vi "AO_Volt_and_Curr.vi"(6 "Curnt_Value":dbl[](array[numeric]) format="%0.2f", 7 "Volt_Value":dbl[](array[numeric]) format="%0.2f", 9 "Current Channel":string[](array[string]), 10 "Volt Channel":string[](array[string])) -> (0 "error out":errorcluster)   [LabVIEW 2017]
uses:
  <vilib>/DAQmx/write.llb/DAQmx Write (Analog 1D DBL NChan 1Samp).vi
  <vilib>/DAQmx/create/channels.llb/DAQmx Create Channel (AO-Voltage-Basic).vi
  <vilib>/DAQmx/miscellaneous.llb/DAQmx Fill In Error Info.vi
  <vilib>/DAQmx/create/channels.llb/DAQmx Create Channel (AO-Current-Basic).vi
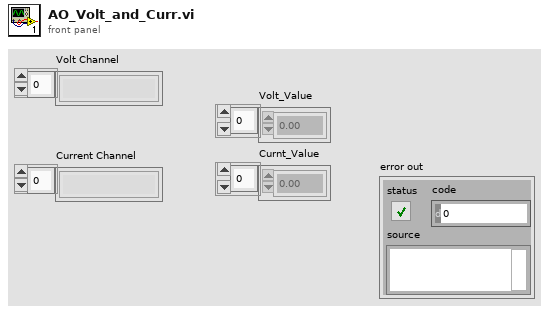
[diagram p1: front panel]
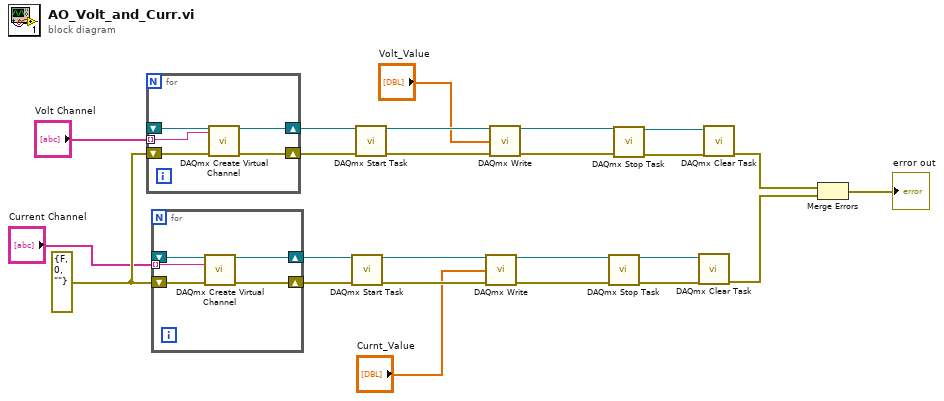
[diagram p0: block diagram]
diagram:
  w4 = errorcluster {"status"=FALSE, "code"=0, "source"=""} ("error out")
  n1 = for {
    shift-right: [w29] -> w24
    shift-left: _ -> [w27]
    shift-right: [w28] -> w23
    shift-left: w4 -> [w26]
    tunnel: "Volt Channel" -> [w25] mode=indexing
    n2 = call-poly <vilib>:"DAQmx Create Virtual Channel.vi"("task in"=w27, "physical channels"=w25, "error in"=w26) -> ("task out"=w29:refnum<k21>, "error out"=w28:errorcluster)  [unwired: 11 in]
  }
  n3 = for {
    shift-right: [w34] -> w18
    shift-left: _ -> [w32]
    shift-right: [w33] -> w17
    shift-left: w4 -> [w31]
    tunnel: "Current Channel" -> [w30] mode=indexing
    n4 = call-poly <vilib>:"DAQmx Create Virtual Channel.vi"("task in"=w32, "physical channels"=w30, "error in"=w31) -> ("task out"=w34:refnum<k21>, "error out"=w33:errorcluster)  [unwired: 11 in]
  }
  n5 = call <vilib>:"DAQmx Start Task.vi"("task/channels in"=w18, "error in"=w17) -> ("task out"=w19:refnum<k21>, "error out"=w20:errorcluster)  [unwired: 12 in]
  n6 = call <vilib>:"DAQmx Start Task.vi"("task/channels in"=w24, "error in"=w23) -> ("task out"=w22:refnum<k21>, "error out"=w21:errorcluster)  [unwired: 12 in]
  n7 = call-poly <vilib>:"DAQmx Write.vi"("task/channels in"=w19, "data"="Curnt_Value", "error in"=w20) -> ("task out"=w10:refnum<k21>, "error out"=w9:errorcluster)  [unwired: 10 in, 1 out]
  n8 = call-poly <vilib>:"DAQmx Write.vi"("task/channels in"=w22, "data"="Volt_Value", "error in"=w21) -> ("task out"=w16:refnum<k21>, "error out"=w15:errorcluster)  [unwired: 10 in, 1 out]
  n9 = call <vilib>:"DAQmx Stop Task.vi"("task/channels in"=w10, "error in"=w9) -> ("task out"=w12:refnum<k21>, "error out"=w11:errorcluster)  [unwired: 12 in]
  n10 = call <vilib>:"DAQmx Stop Task.vi"("task/channels in"=w16, "error in"=w15) -> ("task out"=w13:refnum<k21>, "error out"=w14:errorcluster)  [unwired: 12 in]
  n11 = call <vilib>:"DAQmx Clear Task.vi"("task in"=w12, "error in"=w11) -> ("error out"=w7:errorcluster)  [unwired: 13 in]
  n12 = call <vilib>:"DAQmx Clear Task.vi"("task in"=w13, "error in"=w14) -> ("error out"=w8:errorcluster)  [unwired: 13 in]
  n13 = Merge Errors(w8, w7) -> (→"error out":errorcluster)
